vi "CSM - Remove Loop Tag to Break.vi"(11 "Remaining States":string) -> (3 "States":string)   [LabVIEW 2014, in "CSM Loop Support.lvlib"]
uses:
  CSM Loop Support.lvlib
  Communicable State Machine.lvlib
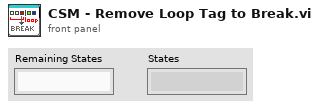
[diagram p1: front panel]
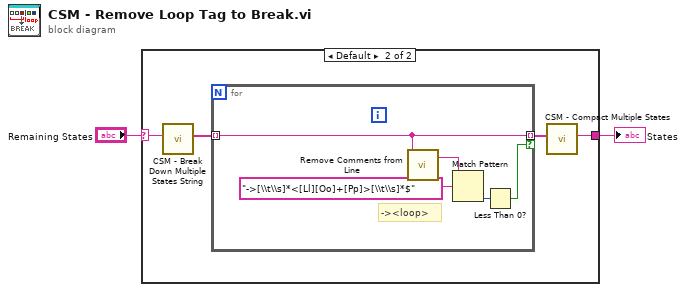
[diagram p0: block diagram]
diagram:
  n1 = case shown="Default" "Remaining States" {
    selector: "Remaining States" -> [w3 w4]
    tunnel: [w3 w5] -> w2
    frame "" {
    }
    frame Default {
      n2 = call "CSM - Break Down Multiple States String.vi"("States"=w4) -> ("Multiple States"=w7:string[])  [unwired: 10 in]
      n3 = for {
        tunnel: [w9] -> w6 mode=indexing if=w10
        tunnel: w7 -> [w9] mode=indexing
        # "-><loop>"
        n4 = call "Remove Comments from Line.vi"("single-line text"=w9) -> ("single-line text without comments"=w8:string)  [unwired: 2 in]
        n5 = Match Pattern(string=w8, regular expression="->[\\t\\s]*<[Ll][Oo]+[Pp]>[\\t\\s]*$") -> (offset past match=w11:i32)  [unwired: 1 in, 3 out]
        n6 = Less Than 0?(x=w11) -> (x < 0?=w10:bool)
      }
      n7 = call "CSM - Compact Multiple States.vi"("Multiple States"=w6) -> ("States"=w5:string)  [unwired: 9 in]
    }
  }
  "States" <- w2
